vi "WF phase diversity_MATLAB_Correction_loop_AndorSDK_imq_NotOverwriteFolder.vi"() -> ()   [LabVIEW 2018]
uses:
  <userlib>/WaveKit.lib/Controls/Wavefront Corrector states - ONE.ctl
  <userlib>/WaveKit.lib/Classes/WavefrontCorrector/WavefrontCorrector.lvclass
  <userlib>/WaveKit.lib/Classes/WavefrontCorrectorSet/WavefrontCorrectorSet.lvclass
  <vilib>/Analysis/1siggen.llb/Ramp Pattern by Samples.vi
  <vilib>/Utility/file.llb/Read From Spreadsheet File (DBL).vi
  <vilib>/Analysis/1siggen.llb/Ramp Pattern by Delta.vi
  <vilib>/Analysis/NI_AALBase.lvlib
panel:
  in  "Tab Control":T1(tab)
  in  "Offset command file":path=path "D:/SystemAlignment/system_aberration_20200627.dat"
  in  "Initial haso file":path=path "D:/SystemAlignment/system_aberration_residual_20200627.has"
  out "# of Phase":i32
  in  "DM configuration file":path=path "C:/Program Files (x86)/Imagine Optic/Configuration Files/WaveFrontCorrector_mirao52-e_0326.dat"
  out "DM Initial State":T2[](array[typedef])
  out "DM ActuatorsNumber":i32
  out "Error out":errorcluster
  in  "Error in":errorcluster
  in  "EMCCD trigger port":tag="Dev1/port0/line0"
  in  "Cooler set to Temperature":i32=-60
  in  "Trigger":u32(ring)=1 items=["Internal", "External"]
  out "Return from CheckTimings":u32
  out "Calculated Exposure Value":sgl format="%.2f"
  out "Return from SetTemperature":u32
  out "Cooling":i32
  out "Return from Initialize":u32
  out "Detector X Pixels":i32
  out "Detector Y Pixels":i32
  in  "Initialize EMCCD?":bool=TRUE
  in  "Turn off EMCCD when finished?":bool
  in  "Initial Zer coeff":dbl[](array[numeric])=[0.2, 0.2]
  in  "Initial Zer index":dbl[](array[numeric])=[4.0, 5.0]
  out "Initial Zer coeff\nRandomly generated":dbl[](array[numeric])
  out "Initial Zer index (starting from 4)\nrandomly generated":dbl[](array[numeric])
  in  "aberration tolerance":dbl=0.1 format="%#_13g"
  in  "aberration threshold":dbl=0.25 format="%#_13g"
  in  "?":enum16{"input manually ", "randomly generated"}(ring)
  in  "max random order":i64=9
  in  "NOT YET: Data Acquisition Iteration #":i32=1
  in  "Zern index in 2":i32[](array[numeric])=[3, 4, 5, 6, 7, 8]
  in  "Zern coef in 2":sgl[](array[numeric])=[0.2, 0.5, 0.0, 0.0, 0.0, 0.0]
  in  "Zern index in 3":i32[](array[numeric])=[3, 4, 5, 6, 7, 8]
  in  "Zern coef in 3":sgl[](array[numeric])=[0.2, 0.0, 0.0, 0.0, 0.0, 0.0]
  in  "Zern index in 4":i32[](array[numeric])=[3, 4, 5, 6, 7, 8]
  in  "Zern coef in 4":sgl[](array[numeric])=[0.2, 0.0, 0.0, 0.0, 0.0, 0.0]
  in  "Zern index in 5":i32[](array[numeric])=[3, 4, 5, 6, 7, 8]
  in  "Zern coef in 5":sgl[](array[numeric])=[0.0, 0.0, 0.0, 0.0, 0.0, -0.2]
  in  "Andor Picture/notes save to path":path=path "D:/YD/test/test1"
  in  "base name":string="beads_test"
  in  "Pics/phase":dbl=2.0
  in  "camera exposure time (s)":string="0.02"
  in  "# of Phase":i32=5
  in  "COMMAND matrix path":path=path "D:/SystemAlignment/CM_20200711_0p5x6.aomc"
  in  "488 shutter":refnum<k7>(container)
  in  "?":bool
  out "phase diversity file name":string
  out "Corrected Picture name":string
  in  "Use GPU":bool=TRUE
  in  "Show Recon":bool=TRUE
  in  "Show Input":bool
  in  "Background Value":u32=290
  in  "Crop Size of image":u32=512
  in  "Gamma Value":dbl=1e-06
  in  "Iteration Number":u32=10
  in  "Zernike Order":u32=15
  in  "Number for average":u32=2
  in  "Run MATLAB or correction?":bool=TRUE
  in  "Keep Reconstructed Defocus component?":bool
  in  "Metrics Type":T3(ring)=enum."norm DCT  - spectral domain 3: 0~r0"
  in  "number of phase div image":dbl(ring)=2.0 items=["adding by step of 1 image"=1.0, "jump to 3 images"=0.9, "jump to 4 images"=2.0, "jump to 5 images"=2.9]
  # "priority:\n1, flip, done by Min on 20200731? \n2, organize\n3, new matlab PD code\n4. isolate shutdown\n\n\n\n2 PhasDiv first\nif not, take 3 more or start over 5\n\n??: random iteration work??\n\nadd preview"
  # "Cooler is off for testing"
  # "If Pics/phase is 2:\npicture order:\n\noffset+aberr *2\nphase diversity *8\n\nground truth *1\noffset+aberr *1\ncorrected *2 but the last one cannot be seen in imagej"
  # "Randomly Generate Initial Zernike, enter here:"
  # "Manually input, enter here:"
  # "Andor Camera Settings"
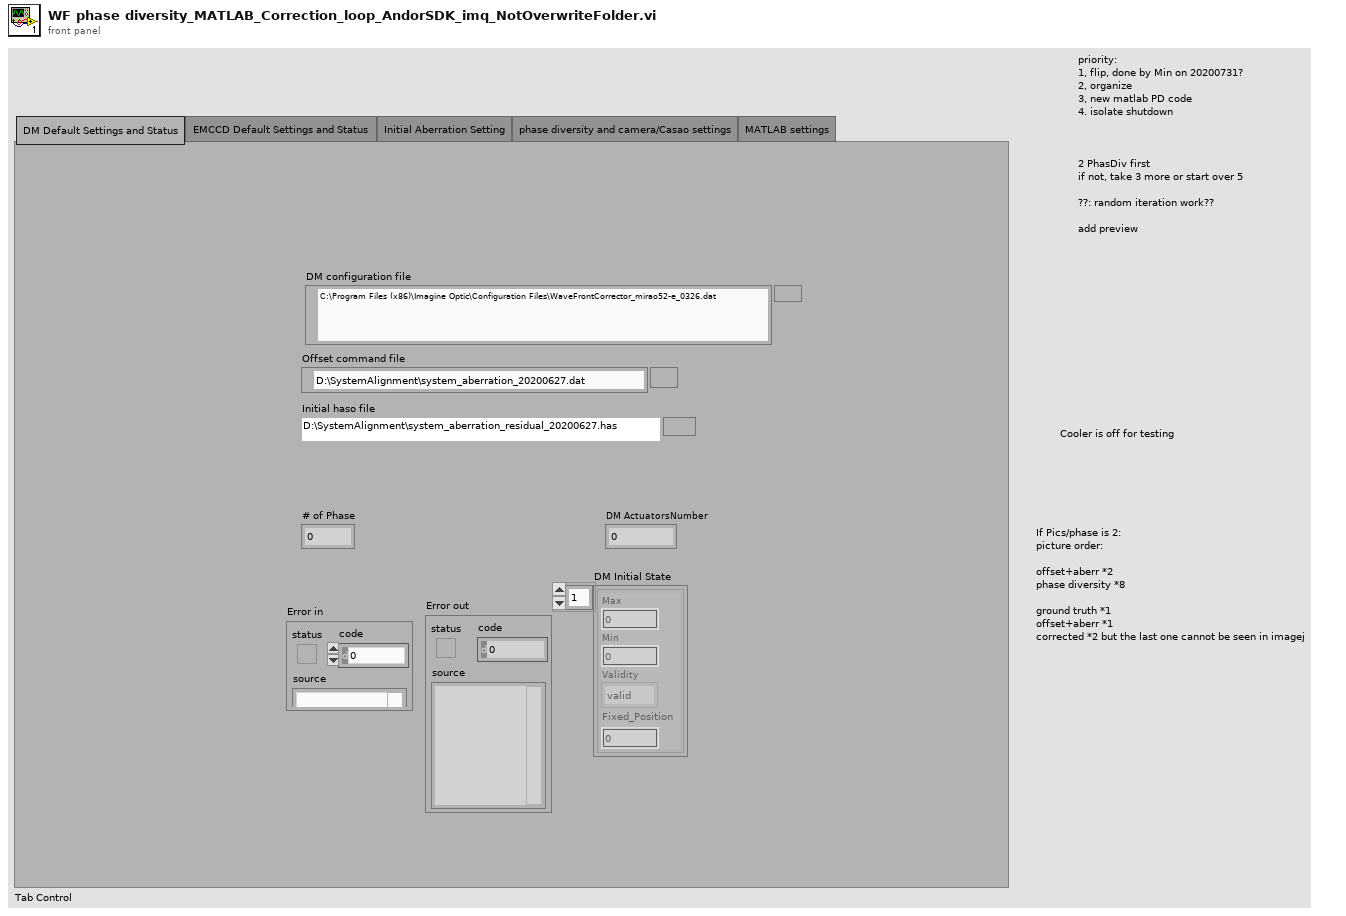
[diagram p1: front panel]
types:
  T1 = enum32{"DM Default Settings and Status", "EMCCD Default Settings and Status ", "Initial Aberration Setting", "phase diversity and camera/Casao settings", "MATLAB settings"}
  T2 = typedef "Wavefront Corrector states - ONE.ctl" = cluster{"Max":sgl, "Min":sgl, "Validity":enum16{"valid", "fixed", "invalid"}, "Fixed_Position":sgl}
  T3 = enum16{" ", "max intensity", "mean intensity", "RMS contrast", "sharpness - image domain", "sharpness - spectral domain 1: 0~r0", "sharpness - spectral domain 2: 0.1*r0~0.5*r0", "norm DCT  - spectral domain 3: 0~r0"}
  T4 = typedef "Error Code Enum typedef.ctl" = enum32{"N/A (0)", "DRV_ERROR_CODES", "DRV_SUCCESS", "DRV_VXDNOTINSTALLED", "DRV_ERROR_SCAN", "DRV_ERROR_CHECK_SUM", "DRV_ERROR_FILELOAD", "DRV_UNKNOWN_FUNC", "DRV_ERROR_VXD_INIT", "DRV_ERROR_ADDRESS", "DRV_ERROR_PAGELOCK", "DRV_ERROR_PAGEUNLOCK", "DRV_ERROR_BOARDTEST", "DRV_ERROR_ACK", "DRV_ERROR_UP_FIFO", "DRV_ERROR_PATTERN", "N/A (16)", "DRV_ACQUISITION_ERRORS", "DRV_ACQ_BUFFER", "DRV_ACQ_DOWNFIFO_FULL", "DRV_PROC_UNKONWN_INSTRUCTION", "DRV_ILLEGAL_OP_CODE", "DRV_KINETIC_TIME_NOT_MET", "DRV_ACCUM_TIME_NOT_MET", "DRV_NO_NEW_DATA", "N/A (25)", "DRV_SPOOLERROR", "N/A (27)", "N/A (28)", "N/A (29)", "N/A (30)", "N/A (31)", "N/A (32)", "DRV_TEMPERATURE_CODES", "DRV_TEMPERATURE_OFF", "DRV_TEMPERATURE_NOT_STABILIZED", "DRV_TEMPERATURE_STABILIZED", "DRV_TEMPERATURE_NOT_REACHED", "DRV_TEMPERATURE_OUT_RANGE", "DRV_TEMPERATURE_NOT_SUPPORTED", "DRV_TEMPERATURE_DRIFT", "N/A (41)", "N/A (42)", "N/A (43)", "N/A (44)", "N/A (45)", "N/A (46)", "N/A (47)", "N/A (48)", "DRV_GENERAL_ERRORS", "DRV_INVALID_AUX", "DRV_COF_NOTLOADED", "DRV_FPGAPROG", "DRV_FLEXERROR", "DRV_GPIBERROR", "N/A (55)", "N/A (56)", "N/A (57)", "N/A (58)", "N/A (59)", "N/A (60)", "N/A (61)", "N/A (62)", "N/A (63)", "DRV_DATATYPE", "DRV_DRIVER_ERRORS", "DRV_P1INVALID", "DRV_P2INVALID", "DRV_P3INVALID", "DRV_P4INVALID", "DRV_INIERROR", "DRV_COFERROR", "DRV_ACQUIRING", "DRV_IDLE", "DRV_TEMPCYCLE", "DRV_NOT_INITIALIZED", "DRV_P5INVALID", "DRV_P6INVALID", "DRV_INVALID_MODE", "DRV_INVALID_FILTER", "DRV_I2CERRORS", "DRV_I2CDEVNOTFOUND", "DRV_I2CTIMEOUT", "DRV_P7INVALID", "N/A (84)", "N/A (85)", "N/A (86)", "N/A (87)", "N/A (88)", "N/A (89)", "DRV_IOCERROR", "DRV_VRMVERSIONERROR"}
  T5 = typedef "NI_Matrix.lvlib/RealMatrix.ctl" = dbl[][]
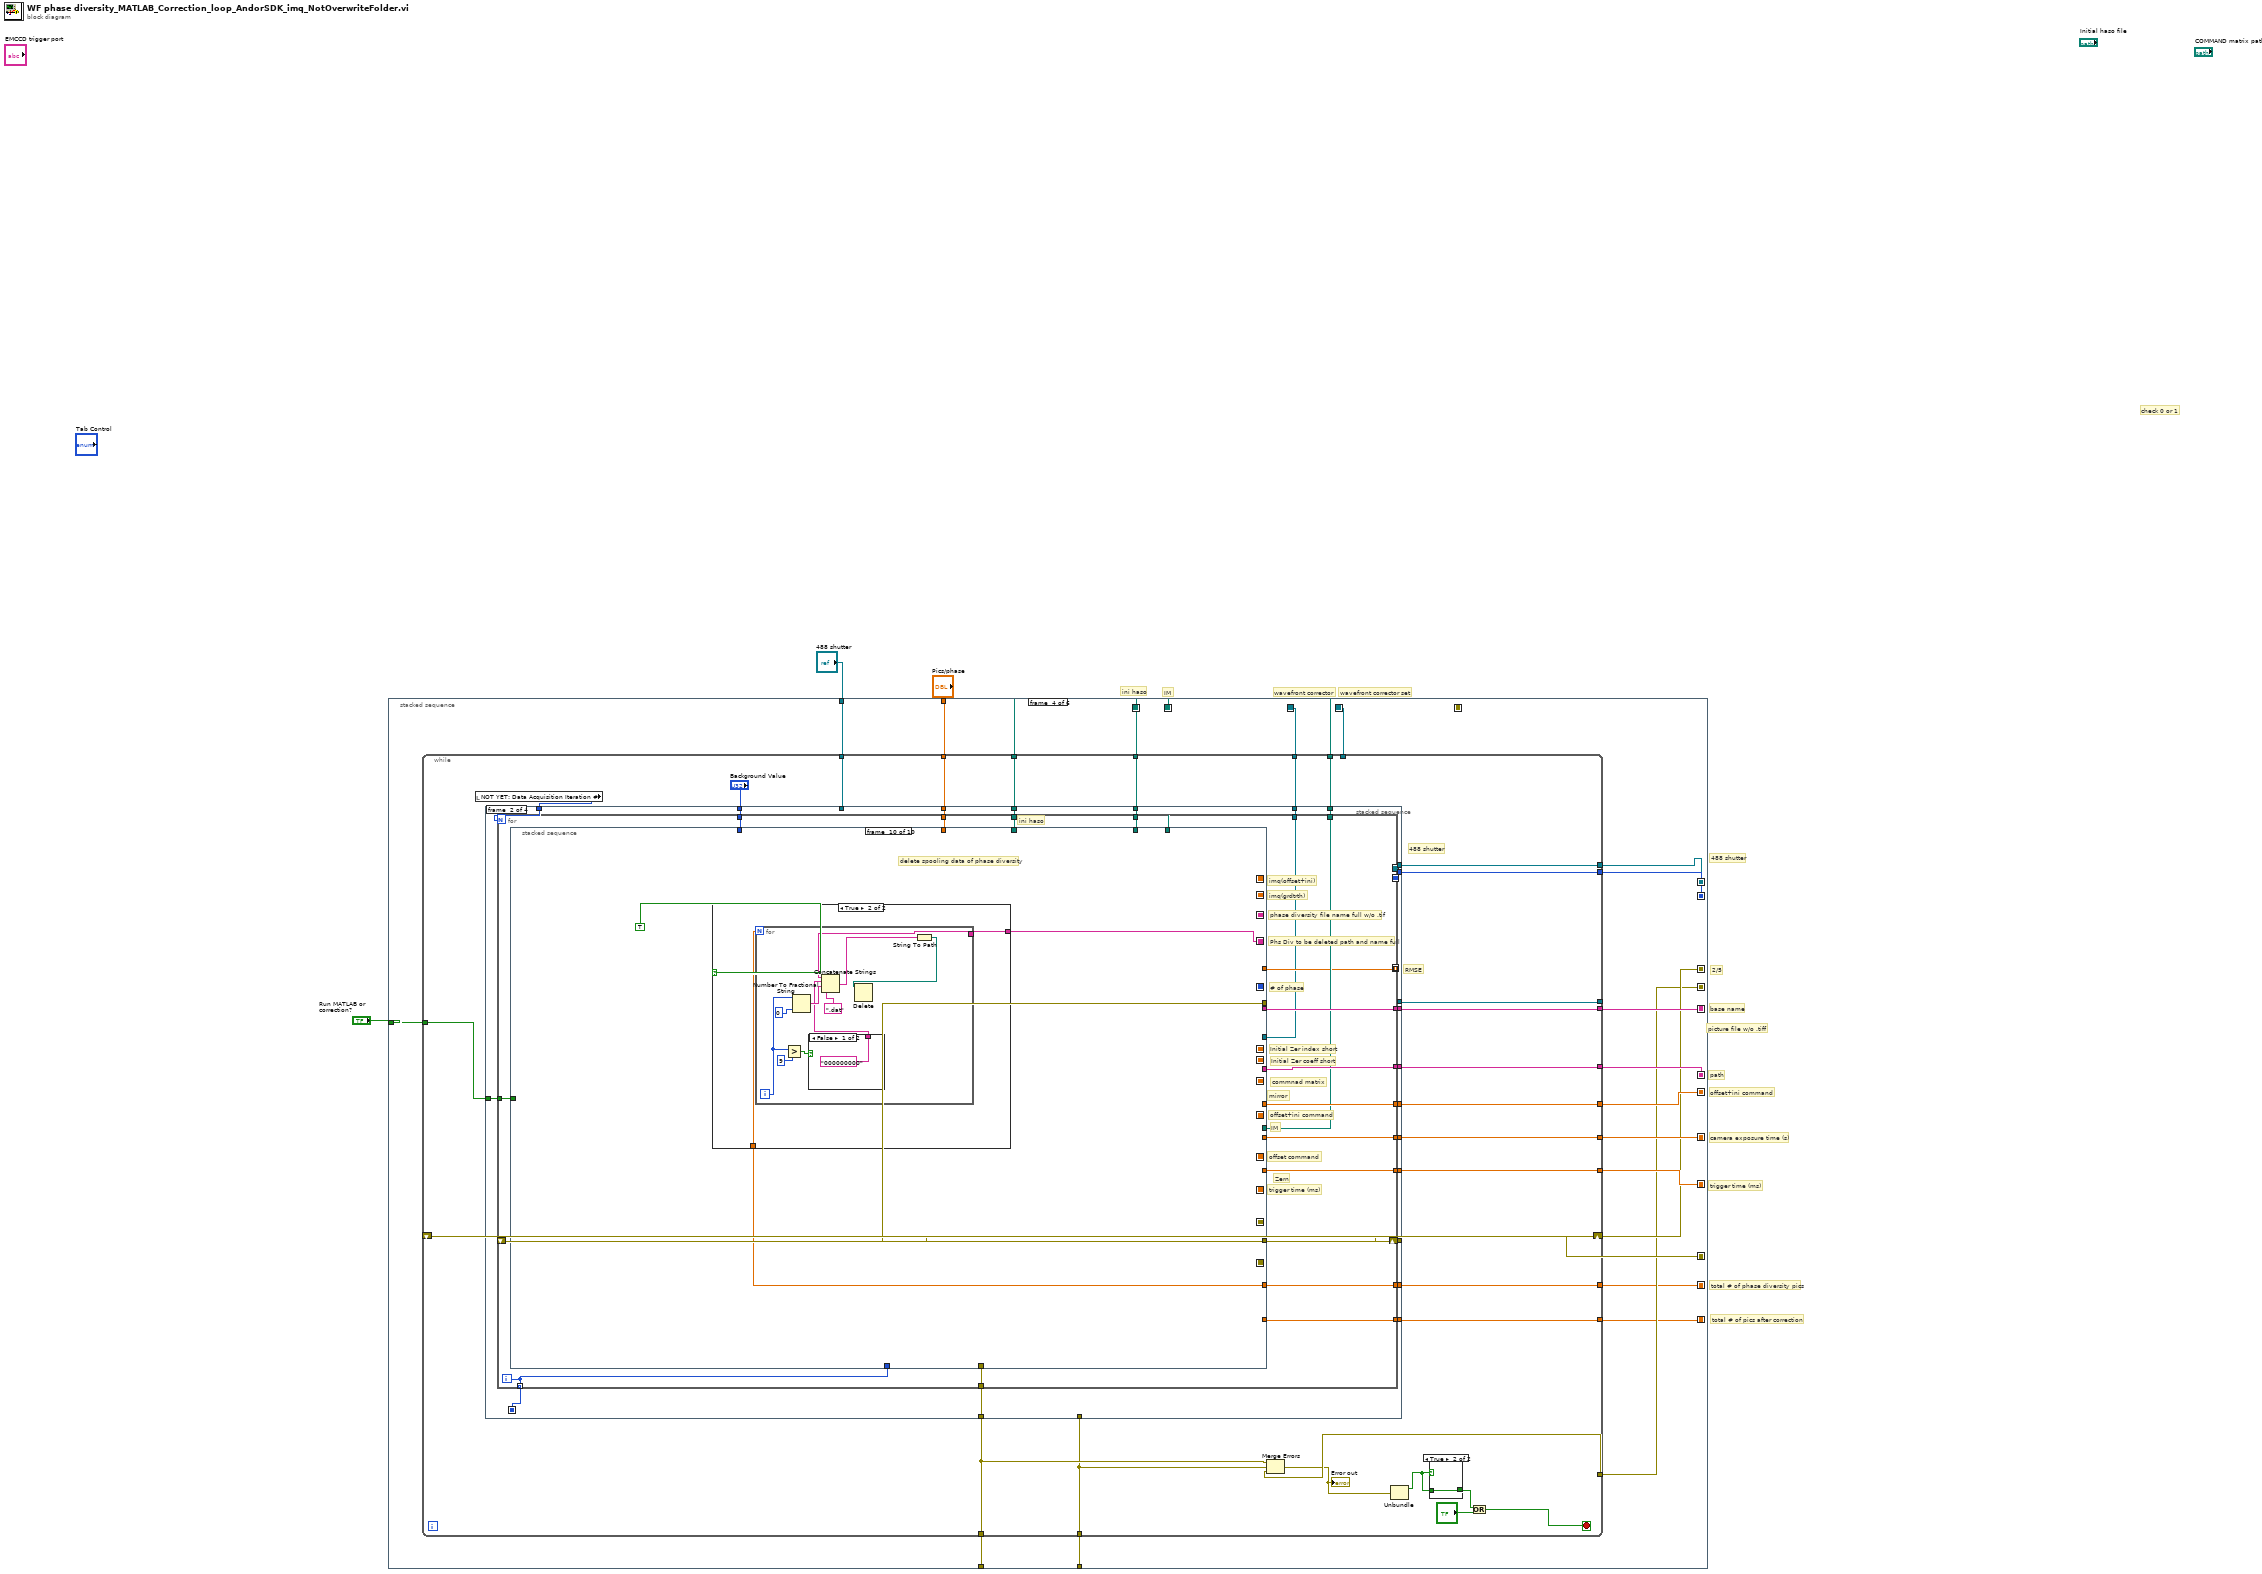
[diagram p0: block diagram]
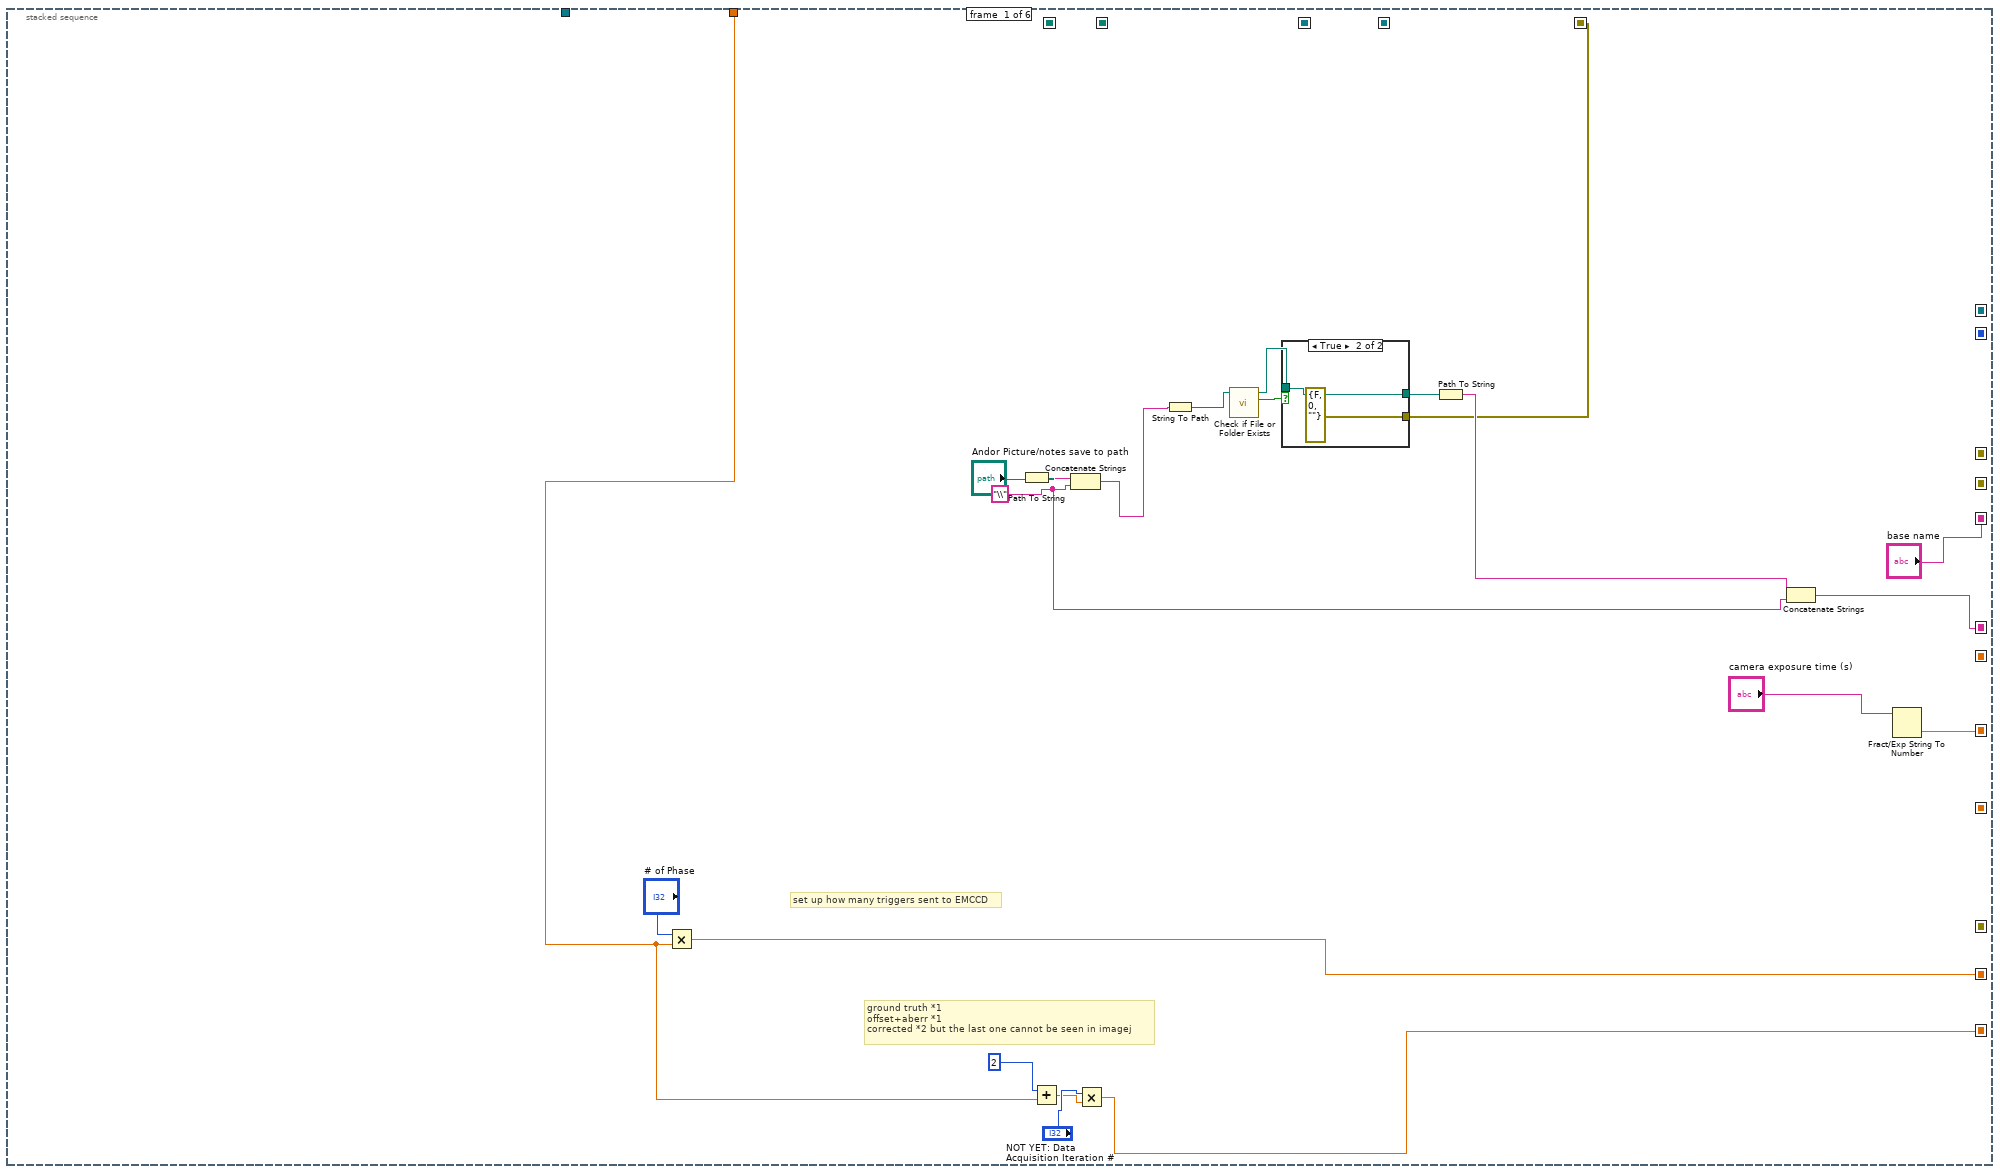
[diagram p2: hidden frame]
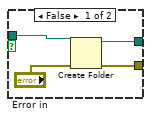
[diagram p3: hidden frame]
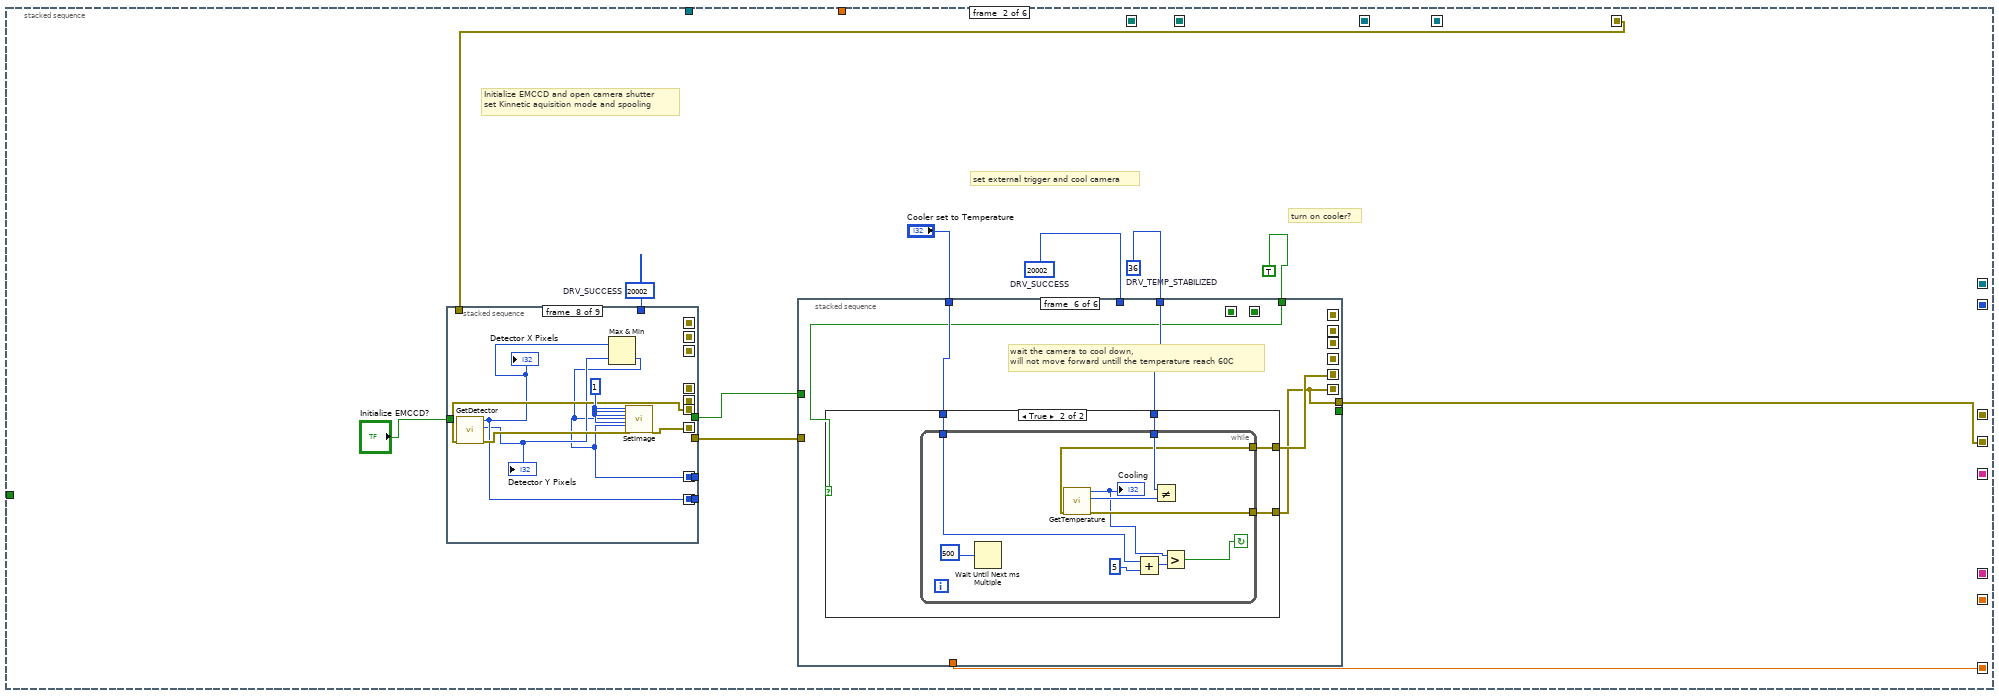
[diagram p4: hidden frame]
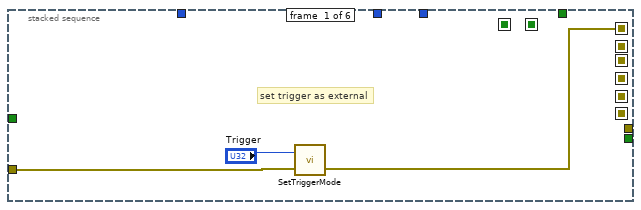
[diagram p5: hidden frame]
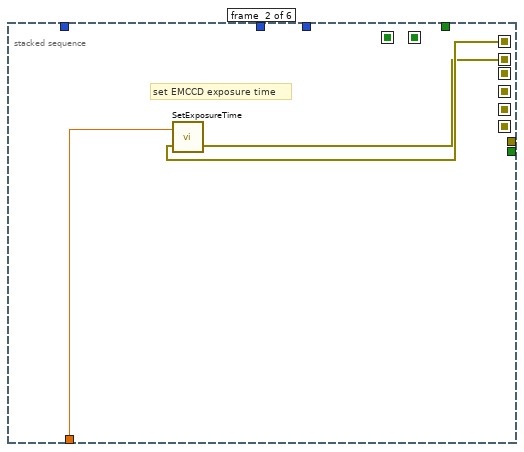
[diagram p6: hidden frame]
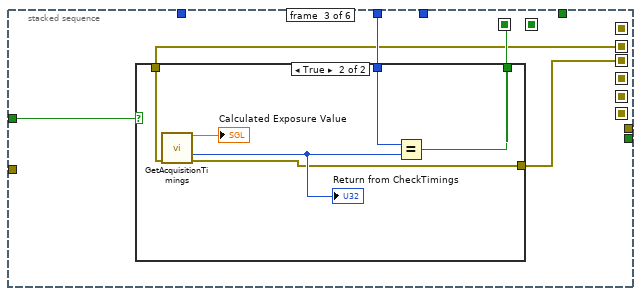
[diagram p7: hidden frame]
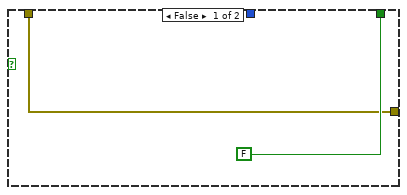
[diagram p8: hidden frame]
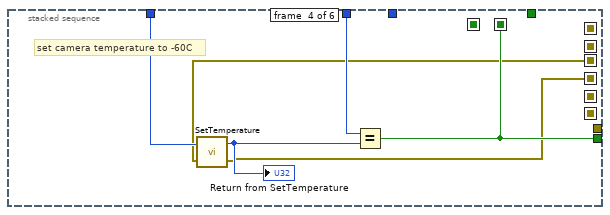
[diagram p9: hidden frame]
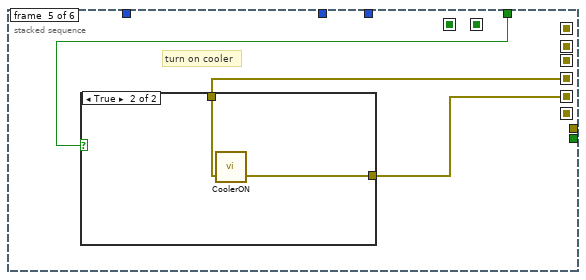
[diagram p10: hidden frame]
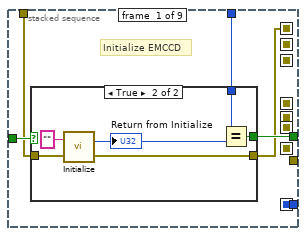
[diagram p13: hidden frame]
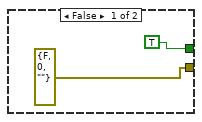
[diagram p14: hidden frame]
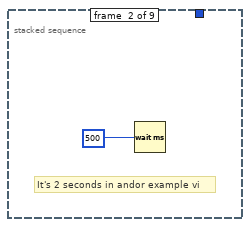
[diagram p15: hidden frame]
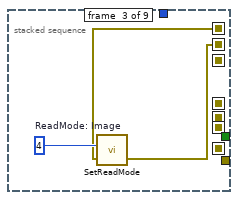
[diagram p16: hidden frame]
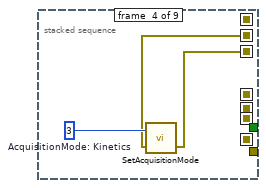
[diagram p17: hidden frame]
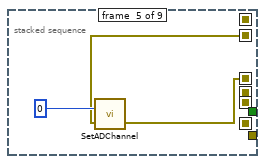
[diagram p18: hidden frame]
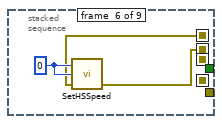
[diagram p19: hidden frame]
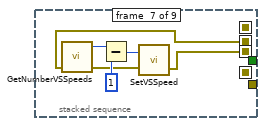
[diagram p20: hidden frame]
diagram:
  # "2/5"
  # "total # of phase diversity pics"
  # "picture file w/o .tiff"
  # "total # of pics after correction"
  # "wavefront corrector set"
  # "wavefront corrector"
  # "488 shutter"
  # "trigger time (ms)"
  # "offset+ini command"
  # "camera exposure time (s)"
  # "IM"
  # "ini haso"
  # "path"
  # "base name"
  # "check 0 or 1"
  n1 = stacked-sequence {
    seq-local: [w5 _ _ _ _ _] -> [_ _ _ w174 _ _]
    seq-local: ["base name" _ _ _ _ _] -> [_ _ _ w173 _ _]
    seq-local: [_ _ w154 _ _ _] -> [_ _ _ w155 _ _]
    seq-local: [_ _ w153 _ _ _] -> [_ _ _ w168 _ _]
    seq-local: [w19 _ _ _ _ _] -> [_ w34 _ w172 _ _]
    seq-local: [_ _ w139 _ _ _] -> [_ _ _ w160 _ _]
    seq-local: [_ _ _ w171 _ _] -> [_ _ _ _ _ _]
    seq-local: [_ _ _ w170 _ _] -> [_ _ _ _ _ _]
    seq-local: [_ _ _ w169 _ _] -> [_ _ _ _ _ w788]
    seq-local: [_ _ _ w163 _ _] -> [_ _ _ _ _ _]
    seq-local: [_ _ _ w166 _ _] -> [_ _ _ _ _ _]
    seq-local: [_ _ w138 _ _ _] -> [_ _ _ w161 _ w790]
    seq-local: [_ _ w137 _ _ _] -> [_ _ _ w159 _ w789]
    seq-local: [w16 _ _ _ _ _] -> [_ _ _ w156 _ _]
    seq-local: [_ w35 _ _ _ _] -> [_ _ w136 w158 _ _]
    seq-local: [w15 _ _ _ _ _] -> [_ _ _ w157 _ _]
    seq-local: [w4 _ _ _ _ _] -> [_ w31 _ _ _ _]
    tunnel: "Pics/phase" -> [w13 _ _ w175 _ _]
    tunnel: "Run MATLAB or correction?" -> [_ _ _ w167 _ _]
    tunnel: [_ _ _ w165 _ _] -> _
    tunnel: [_ _ _ w164 _ _] -> _
    tunnel: "488 shutter" -> [_ _ _ w162 _ w791]
    frame #0 {
      w6 = "\\"
      # "set up how many triggers sent to EMCCD"
      # "ground truth *1\noffset+aberr *1\ncorrected *2 but the last one cannot be seen in imagej"
      n2 = Multiply(x="# of Phase", y=w13) -> (x*y=w15:dbl)
      n3 = Path To String(path="Andor Picture/notes save to path") -> (string=w21:string)
      n4 = Add(x=2, y=w13) -> (x+y=w17:dbl)
      n5 = Concatenate Strings(w21, w6) -> (w8:string)
      n6 = Multiply(x="NOT YET: Data Acquisition Iteration #", y=w17) -> (x*y=w16:dbl)
      n7 = String To Path(string=w8) -> (path=w12:path)
      n8 = call <vilib>:"Check if File or Folder Exists.vi"("path"=w12) -> ("file or folder exists?"=w10:bool, "dup path"=w11:path)  [unwired: 8 in, 1 out]
      n9 = case shown="True" w10 {
        tunnel: w11 -> [w28 w30]
        tunnel: [w27 w30] -> w9
        tunnel: [w25 errorcluster {"status"=FALSE, "code"=0, "source"=""} ("Error in 3")] -> w4
        frame False {
          n10 = Create Folder(path (use dialog)=w28, error in="Error in") -> (created path=w27:path, error out=w25:errorcluster)  [unwired: 1 in, 1 out]
        }
        frame True {
        }
      }
      n11 = Path To String(path=w9) -> (string=w7:string)
      n12 = Concatenate Strings(w7, w6) -> (w5:string)
      n13 = Fract/Exp String To Number(string="camera exposure time (s)") -> (number=w19:dbl)  [unwired: 3 in, 1 out]
    }
    frame #1 {
      w37 = 36  # DRV_TEMP_STABILIZED
      w39 = 20002  # DRV_SUCCESS
      w41 = 20002  # DRV_SUCCESS
      # "turn on cooler?"
      # "set external trigger and cool camera"
      # "Initialize EMCCD and open camera shutter\nset Kinnetic aquisition mode and spooling"
      n14 = stacked-sequence {
        seq-local: [_ _ _ _ _ _ _ w125 _] -> [_ _ _ _ _ _ _ _ _]
        seq-local: [_ _ _ _ _ _ _ w127 _] -> [_ _ _ _ _ _ _ _ _]
        seq-local: [w95 _ _ _ _ _ _ _ _] -> [_ _ w108 _ _ _ _ _ _]
        seq-local: [_ _ w107 _ _ _ _ _ _] -> [_ _ _ w111 _ _ _ _ _]
        seq-local: [_ _ _ w110 _ _ _ _ _] -> [_ _ _ _ w113 _ _ _ _]
        seq-local: [_ _ _ _ w114 _ _ _ _] -> [_ _ _ _ _ w117 _ _ _]
        seq-local: [_ _ _ _ _ w116 _ _ _] -> [_ _ _ _ _ _ w121 _ _]
        seq-local: [_ _ _ _ _ _ w119 _ _] -> [_ _ _ _ _ _ _ w130 _]
        seq-local: [_ _ _ _ _ _ _ w128 _] -> [_ _ _ _ _ _ _ _ w133]
        tunnel: w41 -> [w97 _ _ _ _ _ _ _ _]
        tunnel: [w96 _ _ _ _ _ _ _ _] -> w40
        tunnel: [_ _ _ _ _ _ _ w125 _] -> _
        tunnel: [_ _ _ _ _ _ _ w127 _] -> _
        tunnel: [_ _ _ _ _ _ _ _ w132] -> w36
        tunnel: "Initialize EMCCD?" -> [w94 _ _ _ _ _ _ _ _]
        tunnel: w31 -> [w93 _ _ _ _ _ _ _ _]
        frame #0 {
          # "Initialize EMCCD"
          n15 = case shown="True" w94 {
            tunnel: w97 -> [_ w103]
            tunnel: [TRUE w102] -> w96
            tunnel: [errorcluster {"status"=FALSE, "code"=0, "source"=""} ("Error in 2") w101] -> w95
            tunnel: w93 -> [_ w100]
            frame False {
            }
            frame True {
              n16 = call <userlib>:"Initialize.vi"("error in (no error)"=w100, "directory (\"\")"="" ("directory (\"\")")) -> ("error out"=w101:errorcluster, "DLL error code"=w105:u32)
              "Return from Initialize" <- w105
              n17 = Equal?(x=w103, y=w105) -> (x = y?=w102:bool)
            }
          }
        }
        frame #1 {
          # "It's 2 seconds in andor example vi"
          n18 = Wait (ms)(milliseconds to wait=u32 500) -> ()  [unwired: 1 out]
        }
        frame #2 {
          w109 = u16 4  # ReadMode: Image
          n19 = call <userlib>:"SetReadMode.vi"("error in (no error)"=w108, "mode"=w109) -> ("error out"=w107:errorcluster)  [unwired: 1 out]
        }
        frame #3 {
          w112 = u16 3  # AcquisitionMode: Kinetics
          n20 = call <userlib>:"SetAcquisitionMode.vi"("error in (no error)"=w111, "mode"=w112) -> ("error out"=w110:errorcluster)  [unwired: 1 out]
        }
        frame #4 {
          n21 = call <userlib>:"SetADChannel.vi"("error in (no error)"=w113, "channel"=0) -> ("error out"=w114:errorcluster)  [unwired: 1 out]
        }
        frame #5 {
          w118 = 0
          n22 = call <userlib>:"SetHSSpeed.vi"("error in (no error)"=w117, "index"=w118, "type"=w118) -> ("error out"=w116:errorcluster)  [unwired: 1 in, 1 out]
        }
        frame #6 {
          n23 = call <userlib>:"GetNumberVSSpeeds.vi"("error in (no error)"=w121) -> ("error out"=w120:errorcluster, "number"=w124:i32)  [unwired: 2 in, 1 out]
          n24 = Subtract(x=w124, y=1) -> (x-y=w122:i32)
          n25 = call <userlib>:"SetVSSpeed.vi"("error in (no error)"=w120, "index"=w122) -> ("error out"=w119:errorcluster)  [unwired: 1 out]
        }
        frame #7 {
          w131 = 1
          n26 = call <userlib>:"GetDetector.vi"("error in (no error)"=w130) -> ("error out"=w129:errorcluster, "ypixels"=w126:i32, "xpixels"=w127:i32)  [unwired: 3 in, 1 out]
          "Detector Y Pixels" <- w126
          "Detector X Pixels" <- w127
          n27 = Max & Min(x=w127, y=w126) -> (min(x,y)=w125:i32)  [unwired: 1 out]
          n28 = call <userlib>:"SetImage.vi"("hbin"=w131, "vbin"=w131, "hstart"=w131, "hend"=w125, "vstart"=w131, "vend"=w125, "error in (no error)"=w129) -> ("error out"=w128:errorcluster)  [unwired: 19 in, 1 out]
        }
        frame #8 {
          w134 = 0
          w135 = 1
          n29 = call <userlib>:"SetShutter.vi"("type"=w135, "mode"=w135, "closingtime"=w134, "openingtime"=w134, "error in (no error)"=w133) -> ("error out"=w132:errorcluster)  [unwired: 9 in, 1 out]
        }
      }
      n30 = stacked-sequence {
        seq-local: [_ _ w50 _ _ _] -> [_ _ _ _ _ _]
        seq-local: [_ _ _ w63 _ _] -> [_ _ _ _ _ _]
        seq-local: [w42 _ _ _ _ _] -> [_ w47 _ _ _ _]
        seq-local: [_ w46 _ _ _ _] -> [_ _ w49 _ _ _]
        seq-local: [_ _ w48 _ _ _] -> [_ _ _ w62 _ _]
        seq-local: [_ _ _ w61 _ _] -> [_ _ _ _ w69 _]
        seq-local: [_ _ _ _ w68 _] -> [_ _ _ _ _ w75]
        seq-local: [_ _ _ _ _ w73] -> [_ _ _ _ _ _]
        tunnel: w39 -> [_ _ w52 w66 _ _]
        tunnel: "Cooler set to Temperature" -> [_ _ _ w64 _ w76]
        tunnel: w37 -> [_ _ _ _ _ w77]
        tunnel: [_ _ _ w63 _ _] -> _
        tunnel: w40 -> [_ _ w51 _ _ _]
        tunnel: w36 -> [w43 _ _ _ _ _]
        tunnel: [_ _ _ _ _ w73] -> w35
        tunnel: w34 -> [_ w45 _ _ _ _]
        tunnel: TRUE -> [_ _ _ _ w67 w74]
        frame #0 {
          # "set trigger as external"
          n31 = call <userlib>:"SetTriggerMode.vi"("error in (no error)"=w43, "mode"="Trigger") -> ("error out"=w42:errorcluster)  [unwired: 1 out]
        }
        frame #1 {
          # "set EMCCD exposure time"
          n32 = call <userlib>:"SetExposureTime.vi"("error in (no error)"=w47, "time"=w45) -> ("error out"=w46:errorcluster)  [unwired: 1 out]
        }
        frame #2 {
          n33 = case shown="True" w51 {
            tunnel: w52 -> [_ w58]
            tunnel: [FALSE w60] -> w50
            tunnel: w49 -> [w53 w56]
            tunnel: [w53 w55] -> w48
            frame False {
            }
            frame True {
              n34 = call <userlib>:"GetAcquisitionTimings.vi"("error in (no error)"=w56) -> ("exposure"=→"Calculated Exposure Value":sgl, "DLL error code"=w57:u32, "error out"=w55:errorcluster)  [unwired: 10 in, 2 out]
              "Return from CheckTimings" <- w57
              n35 = Equal?(x=w58, y=w57) -> (x = y?=w60:bool)
            }
          }
        }
        frame #3 {
          # "set camera temperature to -60C"
          n36 = call <userlib>:"SetTemperature.vi"("error in (no error)"=w62, "temperature"=w64) -> ("error out"=w61:errorcluster, "DLL error code"=w65:u32)
          "Return from SetTemperature" <- w65
          n37 = Equal?(x=w66, y=w65) -> (x = y?=w63:bool)
        }
        frame #4 {
          # "turn on cooler"
          n38 = case shown="True" w67 {
            tunnel: w69 -> [w70 w72]
            tunnel: [w70 w71] -> w68
            frame False {
            }
            frame True {
              n39 = call <userlib>:"CoolerON.vi"("error in (no error)"=w72) -> ("error out"=w71:errorcluster)  [unwired: 1 in, 1 out]
            }
          }
        }
        frame #5 {
          # "wait the camera to cool down,\nwill not move forward untill the temperature reach 60C"
          n40 = case shown="True" w74 {
            tunnel: w77 -> [_ w82]
            tunnel: w76 -> [_ w81]
            tunnel: w75 -> [w78 w80]
            tunnel: [w78 w79] -> w73
            frame False {
            }
            frame True {
              n41 = while {
                tunnel: w82 -> [w91]
                tunnel: w81 -> [w86]
                tunnel: w80 -> [w89]
                tunnel: [w88] -> w79
                stop <- w83 continue-if-true
                n42 = Wait Until Next ms Multiple(millisecond multiple=u32 500) -> ()  [unwired: 1 out]
                n43 = call <userlib>:"GetTemperature.vi"("error in (no error)"=w89) -> ("error out"=w88:errorcluster, "status"=w90:T4, "temperature"=w84:i32)  [unwired: 3 in, 1 out]
                "Cooling" <- w84
                n44 = Add(x=w86, y=5) -> (x+y=w85:i32)
                n45 = Not Equal?(x=w91, y=w90) -> ()  [unwired: 1 out]
                n46 = Greater?(x=w84, y=w85) -> (0:w83:bool)
              }
            }
          }
        }
      }
    }
    frame #2 {
      # "Initialize CASAO"
      n47 = call <userlib>:"LVClass_WavefrontCorrectorSet ctor.vi"("WavefrontCorrectorSet in"=refnum<class "WavefrontCorrectorSet.lvclass"> refnum, "PathToWavefrontCorrectorSetupFile"="DM configuration file", "error in (no error)"=w136) -> ("WavefrontCorrectorSet out"=w143:refnum<class "WavefrontCorrectorSet.lvclass">, "error out"=w152:errorcluster)  [unwired: 11 in]
      n48 = call <userlib>:"LVClass_WavefrontCorrector ctor.vi"("WavefrontCorrector in"=refnum<class "WavefrontCorrector.lvclass"> refnum, "PathToWavefrontCorrectorSetupFile"="DM configuration file", "error in (no error)"=w152) -> ("WavefrontCorrector out"=w147:refnum<class "WavefrontCorrector.lvclass">, "error out"=w146:errorcluster)  [unwired: 11 in]
      n49 = call <userlib>:"LVClass_WavefrontCorrector Init.vi"("WavefrontCorrector in"=w147, "set_init_state_from_config_file"=TRUE, "error in (no error)"=w146) -> ("WavefrontCorrector out"=w141:refnum<class "WavefrontCorrector.lvclass">, "error out"=w145:errorcluster)  [unwired: 11 in]
      n50 = call <userlib>:"LVClass_WavefrontCorrectorSet get nb of actuators.vi"("WavefrontCorrectorSet in"=w143, "error in (no error)"=w145) -> ("WavefrontCorrectorSet out"=w137:refnum<class "WavefrontCorrectorSet.lvclass">, "ActuatorsNumber"=→"DM ActuatorsNumber":i32, "error out"=w142:errorcluster)  [unwired: 11 in]
      n51 = call <userlib>:"LVClass_WavefrontCorrector Get Current Preferences.vi"("WavefrontCorrector in"=w141, "error in (no error)"=w142) -> ("WavefrontCorrector out"=w138:refnum<class "WavefrontCorrector.lvclass">, "Mirror preferences.Wavefront Corrector State"=→"DM Initial State":T2[], "error out"=w139:errorcluster)  [unwired: 10 in, 1 out]
      n52 = local read "COMMAND matrix path"() -> (w153:path)
      n53 = local read "Initial haso file"() -> (w154:path)
    }
    frame #3 {
      n54 = while {
        tunnel: w175 -> [w204]
        tunnel: w174 -> [w203]
        tunnel: w173 -> [w202]
        tunnel: w155 -> [w201]
        tunnel: w172 -> [w200]
        tunnel: [w198] -> w171
        tunnel: [w197] -> w170
        tunnel: w168 -> [w195]
        tunnel: w167 -> [w194]
        tunnel: [w193] -> w166
        tunnel: [w192] -> _
        tunnel: [w190] -> w165
        tunnel: [w191] -> w164
        shift-right: [w196] -> w169
        shift-left: w160 -> [w199]
        tunnel: [w189] -> w163
        tunnel: w162 -> [w188]
        tunnel: w161 -> [w187]
        tunnel: w159 -> [_]
        tunnel: w158 -> [w185]
        tunnel: w157 -> [w179]
        tunnel: w156 -> [w178]
        tunnel: w155 -> [w176]
        stop <- w181 stop-if-true
        # "488 shutter"
        # "RMSE"
        n55 = local read "NOT YET: Data Acquisition Iteration #"() -> (w186:i32)
        n56 = stacked-sequence {
          seq-local: [_ w222 _ _] -> [_ _ _ w780]
          seq-local: [_ w221 _ _] -> [_ _ _ _]
          seq-local: [w209 _ _ _] -> [_ _ w776 _]
          seq-local: [w210 _ _ _] -> [_ _ w775 _]
          tunnel: w204 -> [_ w234 _ _]
          tunnel: w203 -> [_ w233 _ w779]
          tunnel: w202 -> [_ w232 _ w778]
          tunnel: w201 -> [_ w231 _ _]
          tunnel: w200 -> [_ w230 _ _]
          tunnel: w199 -> [_ w229 _ _]
          tunnel: [_ w228 _ _] -> w198
          tunnel: [_ w227 _ _] -> w197
          tunnel: [_ w226 _ _] -> w196
          tunnel: w195 -> [_ w225 _ _]
          tunnel: w194 -> [_ w224 _ _]
          tunnel: w186 -> [_ w223 _ _]
          tunnel: [_ _ w774 _] -> w192
          tunnel: [_ _ w773 _] -> w193
          tunnel: [_ _ _ w777] -> w190
          tunnel: [_ w220 _ _] -> w191
          tunnel: [w209 _ _ _] -> w189
          tunnel: w188 -> [w208 _ _ _]
          tunnel: w187 -> [_ w219 _ _]
          tunnel: w179 -> [_ w218 _ _]
          tunnel: w178 -> [_ w217 _ _]
          tunnel: "Background Value" -> [_ w216 _ _]
          tunnel: w176 -> [_ w215 _ _]
          frame #0 {
            # "open the shutter of 488nm laser"
            n57 = property class="MG17Motor"(reference=w208, "HWSerialNum"=85819115.0) -> (reference out=w214:refnum<k7>)  [unwired: 1 in, 1 out]
            n58 = invoke class="MG17Motor" method="StartCtrl"(reference=w214) -> (reference out=w212:refnum<k7>)  [unwired: 2 in, 2 out]
            n59 = invoke class="MG17Motor" method="SC_Enable"(reference=w212, "lChanID"=0) -> (reference out=w209:refnum<k7>, "lChanID"=w210:i32)  [unwired: 2 in, 2 out]
          }
          frame #1 {
            n60 = for {
              N: w223 -> [_]
              tunnel: w234 -> [w253]
              tunnel: w233 -> [w252]
              tunnel: w232 -> [w251]
              tunnel: w231 -> [w250]
              tunnel: w230 -> [w249]
              tunnel: [w247] -> w228
              tunnel: [w246] -> w227
              tunnel: w225 -> [w244]
              tunnel: w224 -> [w243]
              shift-right: [w245] -> w226
              shift-left: w229 -> [w248]
              tunnel: [w242] -> w222 mode=indexing
              tunnel: [w241] -> w221 mode=indexing
              tunnel: [w240] -> w220
              tunnel: w219 -> [w239]
              tunnel: w218 -> [w238]
              tunnel: w217 -> [w237]
              tunnel: w216 -> [w236]
              tunnel: w215 -> [w235]
              i -> [w241]
              # "imq(grdtrth)"
              # "imq(offset+ini)"
              # "Phs Div to be deleted path and name full"
              # "phase diversity file name full w/o .tif"
              # "# of phase"
              # "trigger time (ms)"
              # "offset+ini command"
              # "Initial Zer coeff short"
              # "Initial Zer index short"
              # "mirror"
              # "Zern"
              # "commnad matrix"
              # "ini haso"
              # "IM"
              # "offset command"
              n61 = stacked-sequence {
                seq-local: [_ w265 _ _ _ _ _ _ _ _] -> [_ _ w285 _ w413 _ _ w472 w525 _]
                seq-local: [_ _ w283 _ _ _ _ _ _ _] -> [_ _ _ _ w412 _ _ _ w527 _]
                seq-local: [_ _ w281 _ _ _ _ _ _ _] -> [_ _ _ _ w411 _ _ _ _ _]
                seq-local: [_ _ w274 _ _ _ _ _ _ _] -> [_ _ _ _ w408 _ _ _ _ _]
                seq-local: [w256 _ _ _ _ _ _ _ _ _] -> [_ _ w271 _ _ _ _ _ _ _]
                seq-local: [w255 _ _ _ _ _ _ _ _ _] -> [_ _ w270 _ _ _ _ _ _ _]
                seq-local: [_ _ w269 _ _ _ _ _ _ _] -> [_ _ _ _ _ _ _ w474 w531 _]
                seq-local: [_ _ _ _ w407 _ _ _ _ _] -> [_ _ _ _ _ w457 _ w477 w518 _]
                seq-local: [_ _ _ _ w406 _ _ _ _ _] -> [_ _ _ _ _ _ _ _ w529 _]
                seq-local: [_ _ _ _ _ _ w460 _ _ _] -> [_ _ _ _ _ _ _ _ w521 _]
                seq-local: [_ _ _ w400 _ _ _ _ _ _] -> [_ _ _ _ _ _ _ _ _ w758]
                seq-local: [_ _ _ _ _ _ _ w473 _ _] -> [_ _ _ _ _ _ _ _ _ _]
                seq-local: [_ _ _ _ _ _ _ w471 _ _] -> [_ _ _ _ _ _ _ _ w519 _]
                tunnel: w253 -> [_ _ w278 _ w416 _ _ _ w530 _]
                tunnel: w252 -> [_ _ w279 w403 w415 _ w468 w480 w533 _]
                tunnel: w251 -> [_ _ w280 w402 w414 _ w470 w479 w534 _]
                tunnel: w250 -> [_ _ w277 _ _ _ _ _ w516 _]
                tunnel: w244 -> [_ _ w276 _ w410 _ _ _ _ _]
                tunnel: w249 -> [_ _ _ _ w409 _ _ _ _ _]
                tunnel: w248 -> [_ _ w275 _ _ _ _ _ _ _]
                tunnel: [_ _ _ _ w406 _ _ _ _ _] -> w245
                tunnel: [_ _ w269 _ _ _ _ _ _ _] -> w247
                tunnel: [_ _ _ _ w407 _ _ _ _ _] -> w246
                tunnel: w244 -> [_ _ _ _ _ _ _ _ w532 _]
                tunnel: w243 -> [_ _ _ _ _ _ _ _ w528 _]
                tunnel: w241 -> [_ _ w268 w399 _ _ w469 w478 w517 _]
                tunnel: [_ _ _ _ _ _ _ _ w526 _] -> w242
                tunnel: [_ _ _ _ _ _ _ _ w524 _] -> w240
                tunnel: w239 -> [_ _ _ _ w405 _ _ w476 w523 _]
                tunnel: w238 -> [_ _ _ w404 _ _ _ _ _ w756]
                tunnel: w237 -> [_ _ _ _ _ _ _ _ w522 _]
                tunnel: w236 -> [_ _ _ _ _ _ _ w475 w520 _]
                tunnel: w235 -> [_ _ _ _ _ _ _ _ w515 _]
                frame #0 {
                  # "generate initial aberration (aberr to correct)"
                  n62 = case shown="\"randomly generated\"" "?" {
                    tunnel: ["Initial Zer index" w262] -> w256
                    tunnel: ["Initial Zer coeff" w261] -> w255
                    tunnel: "max random order" -> [_ w260]
                    frame "input manually " {
                    }
                    frame "randomly generated" {
                      # "generate random zernike index and coefficient arrays"
                      n63 = call "Random Aberration Array Generator.vi"("max random order"=w260, "aberration tolerance"="aberration tolerance", "aberration threshold"="aberration threshold") -> ("Zer coeff"=w261:dbl[], "Zer index (starting from 3)"=w262:dbl[])  [unwired: 7 in]
                      "Initial Zer index (starting from 4)\nrandomly generated" <- w262
                      "Initial Zer coeff\nRandomly generated" <- w261
                    }
                  }
                }
                frame #1 {
                  # "read in offset command"
                  n64 = call-poly <vilib>:"Read From Spreadsheet File.vi"("format (%.3f)"="%.8f", "file path (dialog if empty)"="Offset command file") -> ("first row"=w265:dbl[])  [unwired: 5 in, 4 out]
                }
                frame #2 {
                  w290 = 0.0
                  # "ini zern coeff"
                  # "offset+ini command"
                  # "Zern coeff"
                  # "Zern index"
                  # "calculate the command:\nfor phase diversity"
                  n65 = Array Size(array="Zern index in 2") -> (size(s)=w288:i32)
                  n66 = call-poly <vilib>:"Ramp Pattern.vi"("start"=w290, "end"=w290, "samples"=w288) -> ("Ramp Pattern"=w287:dbl[])  [unwired: 7 in, 1 out]
                  n67 = Build Array(w287, "Zern index in 2", "Zern index in 3", "Zern index in 4", "Zern index in 5") -> (w272:T5)
                  n68 = Build Array(w287, "Zern coef in 2", "Zern coef in 3", "Zern coef in 4", "Zern coef in 5") -> (w291:T5)
                  n69 = Transpose Matrix(1:w291) -> (0:w284:T5)
                  n70 = Transpose Matrix(1:w272) -> (0:w282:T5)
                  n71 = Array Size(array=w272) -> (size(s)=w273:i32[])
                  n72 = Index Array(array=w273, index=1) -> (element=w281:i32)
                  "# of Phase" <- w281
                  n73 = stacked-sequence {
                    seq-local: [w300 _ _] -> [_ w318 w384]
                    seq-local: [w301 _ _] -> [_ w312 _]
                    seq-local: [_ w311 _] -> [_ _ w381]
                    seq-local: [w299 _ _] -> [_ w310 _]
                    tunnel: w281 -> [_ w323 _]
                    tunnel: w271 -> [w308 _ _]
                    tunnel: w270 -> [w307 w313 _]
                    tunnel: w276 -> [w306 w320 _]
                    tunnel: w285 -> [w304 _ _]
                    tunnel: w282 -> [_ w322 _]
                    tunnel: w284 -> [_ w321 _]
                    tunnel: w277 -> [w303 w319 _]
                    tunnel: [_ w317 _] -> w283
                    tunnel: w280 -> [_ w315 w382]
                    tunnel: w279 -> [_ w316 w383]
                    tunnel: w278 -> [_ w314 _]
                    tunnel: w275 -> [w302 _ _]
                    tunnel: [_ _ w380] -> w274
                    tunnel: [w300 _ _] -> w269
                    tunnel: w268 -> [_ w309 w378]
                    frame #0 {
                      n74 = call "zern2command_test.vi"("Initial haso file"=w303, "error in (no error)"=w302, "interaction matrix file"=w306, "Zern coef in"=w307, "Zern index in"=w308) -> ("error out"=w301:errorcluster, "Zern coef out"=w299:sgl[], "Offset positions"=w305:sgl[])  [unwired: 4 in]
                      n75 = Add(x=w305, y=w304) -> (x+y=w300:dbl[])
                    }
                    frame #1 {
                      n76 = for {
                        N: w323 -> [w326]
                        tunnel: w322 -> [w339] mode=indexing
                        tunnel: w321 -> [w338] mode=indexing
                        tunnel: w320 -> [w337]
                        tunnel: w319 -> [w336]
                        tunnel: w318 -> [w335]
                        tunnel: [w334] -> w317 mode=indexing
                        tunnel: w316 -> [w333]
                        tunnel: w315 -> [w332]
                        tunnel: w314 -> [w331]
                        tunnel: w313 -> [w330]
                        tunnel: w312 -> [w329]
                        tunnel: [w328] -> w311
                        tunnel: w310 -> [w325]
                        tunnel: w309 -> [w324]
                        i -> [w327]
                        n77 = stacked-sequence {
                          seq-local: [w345 _] -> [_ w364]
                          seq-local: [w341 _] -> [_ w363]
                          tunnel: w339 -> [w354 _]
                          tunnel: w338 -> [w353 _]
                          tunnel: w337 -> [w352 _]
                          tunnel: w336 -> [w351 _]
                          tunnel: w335 -> [w349 _]
                          tunnel: [w348 _] -> w334
                          tunnel: w333 -> [_ w366]
                          tunnel: w332 -> [_ w365]
                          tunnel: w331 -> [_ _]
                          tunnel: w327 -> [w347 _]
                          tunnel: w330 -> [w343 _]
                          tunnel: w329 -> [w342 _]
                          tunnel: [_ w362] -> w328
                          tunnel: w327 -> [_ _]
                          tunnel: w326 -> [_ _]
                          tunnel: w325 -> [w340 _]
                          tunnel: w324 -> [_ w359]
                          frame #0 {
                            n78 = Equal To 0?(x=w347) -> (x = 0?=w346:bool)
                            n79 = call "zern2command_test.vi"("Initial haso file"=w351, "error in (no error)"=w342, "interaction matrix file"=w352, "Zern coef in"=w353, "Zern index in"=w354) -> ("error out"=w341:errorcluster, "Zern coef out"=w344:sgl[], "Offset positions"=w350:sgl[])  [unwired: 4 in]
                            n80 = case shown="False" w346 {
                              tunnel: [w355 w356] -> w345
                              tunnel: w344 -> [w355 _]
                              tunnel: w343 -> [_ _]
                              tunnel: w340 -> [_ w356]
                              frame False {
                              }
                              frame True {
                              }
                            }
                            n81 = Add(x=w349, y=w350) -> (x+y=w348:dbl[])
                          }
                          frame #1 {
                            n82 = Number To Fractional String(number=w359, precision (6)=0) -> (F-format string=w358:string)  [unwired: 2 in]
                            n83 = Concatenate Strings(w366, w365, "_", w358, "_coeff.txt") -> (w374:string)
                            n84 = String To Path(string=w374) -> (path=w373:path)
                            n85 = Open/Create/Replace File(file path (use dialog)=w373, error in=w363, operation (0:open)=3) -> (refnum out=w370:refnum<file>, error out=w371:errorcluster)  [unwired: 3 in, 1 out]
                            n86 = Array To Spreadsheet String(array=w364, 3:"%f") -> (spreadsheet string=w361:string)  [unwired: 1 in]
                            n87 = Set File Position(refnum=w370, from (0:start)=1, error in=w371) -> (refnum out=w368:refnum<file>, error out=w367:errorcluster)  [unwired: 1 in]
                            n88 = Write to Text File(file (use dialog)=w368, text=w361, error in=w367) -> (error out=w362:errorcluster)  [unwired: 1 in, 2 out]
                          }
                        }
                      }
                    }
                    frame #2 {
                      n89 = Number To Fractional String(number=w378, precision (6)=0) -> (F-format string=w377:string)  [unwired: 2 in]
                      n90 = Concatenate Strings(w383, w382, "_", w377, "_IniAbr+offset.txt") -> (w393:string)
                      n91 = String To Path(string=w393) -> (path=w391:path)
                      n92 = Open/Create/Replace File(file path (use dialog)=w391, error in=w381, operation (0:open)=3) -> (refnum out=w388:refnum<file>, error out=w389:errorcluster)  [unwired: 3 in, 1 out]
                      n93 = Array To Spreadsheet String(array=w384, 3:"%f") -> (spreadsheet string=w395:string)  [unwired: 1 in]
                      n94 = Set File Position(refnum=w388, from (0:start)=1, error in=w389) -> (refnum out=w386:refnum<file>, error out=w385:errorcluster)  [unwired: 1 in]
                      n95 = Write to Text File(file (use dialog)=w386, text=w395, error in=w385) -> (error out=w380:errorcluster)  [unwired: 1 in, 2 out]
                    }
                  }
                }
                frame #3 {
                  # "set andor kinetics and spooling, \nstart acquire and wait for the external trigger"
                  n96 = Number To Fractional String(number=w399, precision (6)=0) -> (F-format string=w397:string)  [unwired: 2 in]
                  n97 = Concatenate Strings(w403, w402, "_PhsDiv_ToBeDeleted_", w397) -> (w400:string)
                  n98 = call "SetSpool_WaitForExtTrigger.vi"("path and name"=w400, "Kinetic Series"=w404) -> ()  [unwired: 10 in]
                }
                frame #4 {
                  # "take phase diversity pictures"
                  n99 = for {
                    N: w411 -> [_]
                    tunnel: w416 -> [w427]
                    tunnel: w415 -> [w426]
                    tunnel: w414 -> [w425]
                    tunnel: w410 -> [w424]
                    tunnel: w413 -> [w423]
                    tunnel: w412 -> [w422] mode=indexing
                    tunnel: w409 -> [w421]
                    tunnel: w408 -> [w420]
                    tunnel: [w419] -> w406
                    tunnel: [w418] -> w407
                    tunnel: w405 -> [w417]
                    n100 = stacked-sequence {
                      seq-local: [w428 _] -> [_ w438]
                      tunnel: w427 -> [_ w435]
                      tunnel: w426 -> [_ _]
                      tunnel: w425 -> [_ _]
                      tunnel: w424 -> [_ _]
                      tunnel: w423 -> [_ _]
                      tunnel: w422 -> [w429 _]
                      tunnel: w421 -> [_ w439]
                      tunnel: w420 -> [w430 _]
                      tunnel: [_ w437] -> w419
                      tunnel: [_ w436] -> w418
                      tunnel: w417 -> [w431 _]
                      frame #0 {
                        # "response time of mirror"
                        n101 = call <userlib>:"LVClass_WavefrontCorrector Move to Absolute Position.vi"("WavefrontCorrector in"=w431, "Absolute Positions"=w429, "error in (no error)"=w430) -> ("error out"=w428:errorcluster)  [unwired: 11 in, 1 out]
                        n102 = Add(x=5, y=10) -> (x+y=w432:i32)
                        n103 = Wait (ms)(milliseconds to wait=w432) -> ()  [unwired: 1 out]
                      }
                      frame #1 {
                        n104 = for {
                          N: w435 -> [_]
                          tunnel: w439 -> [w444]
                          tunnel: w438 -> [w443]
                          tunnel: [w442] -> w437
                          tunnel: [w441] -> w436
                          tunnel: w435 -> [w440]
                          n105 = stacked-sequence {
                            tunnel: w444 -> [w449 _]
                            tunnel: w443 -> [w447 _]
                            tunnel: [w446 _] -> w442
                            tunnel: [w445 _] -> w441
                            tunnel: w440 -> [_ w454]
                            frame #0 {
                              n106 = local read "EMCCD trigger port"() -> (w452:tag)
                              n107 = Add(x=w449, y=0.04) -> (x+y=w448:dbl)
                              n108 = Multiply(x=w448, y=1000.0) -> (x*y=w445:dbl)
                              n109 = call "trig EMCCD.vi"("error in (no error)"=w447, "exp time (ms)"=w445, "lines"=w452) -> ("error out"=w446:errorcluster)
                            }
                            frame #1 {
                              n110 = Not Equal?(x=w454, y=1) -> (x != y?=w455:bool)
                              n111 = case shown="True" w455 {
                                frame False {
                                }
                                frame True {
                                n112 = Wait (ms)(milliseconds to wait=50) -> ()  [unwired: 1 out]
                                }
                              }
                            }
                          }
                        }
                      }
                    }
                  }
                }
                frame #5 {
                  # "send out a trigger to EMCCD to end the aquisition."
                  n113 = local read "EMCCD trigger port"() -> (w458:tag)
                  n114 = call "trig EMCCD.vi"("exp time (ms)"=w457, "lines"=w458) -> ()  [unwired: 1 in, 1 out]
                }
                frame #6 {
                  w465 = 0
                  # "save phase diversity pictures:\npictures per phase*number of phases (Eg: 2*5=10 pictures in this file)"
                  n115 = Number To Fractional String(number=w469, precision (6)=w465) -> (F-format string=w464:string)  [unwired: 2 in]
                  n116 = Concatenate Strings(w470, "_", w464) -> (w460:string)
                  "phase diversity file name" <- w460
                  n117 = Concatenate Strings(w460, ".tif") -> (w461:string)
                  n118 = Concatenate Strings(w468, w461) -> (w463:string)
                  n119 = call <userlib>:"SaveAsTiff.vi"("path"=w463, "palette"="C:\\Program Files\\Andor SOLIS\\GREY.PAL", "position"=w465, "type"=1) -> ()  [unwired: 10 in, 2 out]
                }
                frame #7 {
                  # "offset+ini path and name no.tif"
                  # "groundtruth path and name no.tif"
                  # "take a picture of groundtruth and offset+ini abbr, and cal imq for each"
                  n120 = stacked-sequence {
                    seq-local: [w482 _ _ _] -> [_ w495 _ _]
                    seq-local: [_ _ w498 _] -> [_ _ _ w511]
                    tunnel: w480 -> [w487 _ w504 _]
                    tunnel: w479 -> [w486 _ w503 _]
                    tunnel: w478 -> [w485 _ w502 _]
                    tunnel: w477 -> [w484 _ w501 _]
                    tunnel: w474 -> [_ _ w500 _]
                    tunnel: w476 -> [w483 _ w499 _]
                    tunnel: w475 -> [_ w496 _ w514]
                    tunnel: [_ w492 _ _] -> w473
                    tunnel: w472 -> [w481 _ _ _]
                    tunnel: [_ _ _ w509] -> w471
                    frame #0 {
                      # "take a picture of groundtruth"
                      n121 = Number To Fractional String(number=w485, precision (6)=0) -> (F-format string=w488:string)  [unwired: 2 in]
                      n122 = Concatenate Strings(w487, w486, "_grdtrth_", w488) -> (w482:string)
                      n123 = call "Apply DM command and take picture.vi"("WavefrontCorrector in"=w483, "Offset positions"=w481, "trigger time (ms)"=w484, "# of pictures"=1, "path and file name, no .tif at the end"=w482) -> ()  [unwired: 6 in, 1 out]
                    }
                    frame #1 {
                      # "calculate imq of groundtruth"
                      n124 = Concatenate Strings(w495, ".tif") -> (w493:string)
                      n125 = call "MATLAB image quality metrics.vi"("Background Value"=w496, "File Path and Name w/.tif"=w493, "Metrics Type"="Metrics Type") -> ("image quality"=w492:dbl)  [unwired: 8 in]
                    }
                    frame #2 {
                      # "take a picture of offset+ini abbr"
                      n126 = Number To Fractional String(number=w502, precision (6)=0) -> (F-format string=w505:string)  [unwired: 2 in]
                      n127 = Concatenate Strings(w504, w503, "_abbr_", w505) -> (w498:string)
                      n128 = call "Apply DM command and take picture.vi"("WavefrontCorrector in"=w499, "Offset positions"=w500, "trigger time (ms)"=w501, "# of pictures"=1, "path and file name, no .tif at the end"=w498) -> ()  [unwired: 6 in, 1 out]
                    }
                    frame #3 {
                      # "calculate imq of offset+ini"
                      n129 = local read "Metrics Type"() -> (w510:T3)
                      n130 = Concatenate Strings(w511, ".tif") -> (w512:string)
                      n131 = call "MATLAB image quality metrics.vi"("Background Value"=w514, "File Path and Name w/.tif"=w512, "Metrics Type"=w510) -> ("image quality"=w509:dbl)  [unwired: 8 in]
                    }
                  }
                }
                frame #8 {
                  # "run matlab correction?"
                  n132 = case shown="True" w528 {
                    tunnel: w533 -> [_ w556]
                    tunnel: w534 -> [_ w555]
                    tunnel: w532 -> [_ w554]
                    tunnel: w531 -> [_ w553]
                    tunnel: w518 -> [_ w552]
                    tunnel: w530 -> [_ w551]
                    tunnel: w529 -> [_ w550]
                    tunnel: w517 -> [_ w549]
                    tunnel: w527 -> [_ _]
                    tunnel: [0 w548] -> w526
                    tunnel: w525 -> [_ w547]
                    tunnel: [errorcluster {"status"=FALSE, "code"=0, "source"=""} ("Error out 2") w546] -> w524
                    tunnel: w523 -> [_ w545]
                    tunnel: w522 -> [_ w544]
                    tunnel: w521 -> [_ _]
                    tunnel: w520 -> [_ w543]
                    tunnel: w519 -> [_ w540]
                    tunnel: w518 -> [_ w542]
                    tunnel: w517 -> [_ w541]
                    tunnel: w516 -> [_ w538]
                    tunnel: w515 -> [_ w537]
                    frame False {
                    }
                    frame True {
                      # "matlab reconstructed Zern"
                      n133 = stacked-sequence {
                        seq-local: [w569 _ _ _ _ _ _ _ _ _ _] -> [_ _ _ _ _ _ w711 _ _ _ _]
                        seq-local: [w571 _ _ _ _ _ _ _ _ _ _] -> [_ _ _ _ _ _ w707 _ _ _ _]
                        seq-local: [_ _ _ _ w690 _ _ _ _ _ _] -> [_ _ _ _ _ w697 _ _ _ _ _]
                        seq-local: [_ _ w678 _ _ _ _ _ _ _ _] -> [_ _ _ w685 _ _ _ _ _ _ _]
                        seq-local: [_ _ _ w687 _ _ _ _ _ _ _] -> [_ _ _ _ w691 _ _ _ _ _ _]
                        seq-local: [_ w670 _ _ _ _ _ _ _ _ _] -> [_ _ _ _ _ _ _ _ _ _ w745]
                        tunnel: w556 -> [w570 w673 _ _ _ _ _ _ _ w734 _]
                        tunnel: w555 -> [w568 w672 _ _ _ _ _ _ _ w733 _]
                        tunnel: w554 -> [w560 _ _ _ _ _ w710 _ _ _ _]
                        tunnel: w553 -> [w563 _ _ _ w692 _ w709 _ _ _ _]
                        tunnel: w552 -> [_ _ _ w689 _ w699 _ w717 w731 _ _]
                        tunnel: w550 -> [_ _ w679 _ _ _ _ _ _ _ _]
                        tunnel: [_ _ _ w688 _ _ _ _ _ _ _] -> _
                        tunnel: w551 -> [_ _ _ w688 _ _ _ w716 _ _ _]
                        tunnel: w549 -> [w567 w671 _ _ _ _ _ _ _ w735 _]
                        tunnel: [w566 _ _ _ _ _ _ _ _ _ _] -> w548
                        tunnel: w547 -> [_ _ w680 _ _ _ _ _ _ _ _]
                        tunnel: [_ _ _ _ _ _ _ w715 _ _ _] -> w546
                        tunnel: w545 -> [w557 _ w681 _ w693 _ w703 _ _ _ _]
                        tunnel: w544 -> [_ w674 _ _ _ _ _ _ _ _ w743]
                        tunnel: w543 -> [w565 _ _ _ _ _ _ _ _ _ _]
                        tunnel: w542 -> [w562 _ _ _ _ _ _ _ _ _ _]
                        tunnel: w541 -> [w561 _ _ _ _ _ _ _ _ _ _]
                        tunnel: 2 -> [w564 _ _ _ _ _ _ _ _ _ _]
                        tunnel: w540 -> [w559 _ _ _ _ _ _ _ _ _ _]
                        tunnel: w538 -> [w558 _ _ _ _ _ _ _ _ _ _]
                        tunnel: w537 -> [_ _ _ _ _ _ w700 _ _ _ _]
                        frame #0 {
                          n134 = while {
                            tunnel: [w590] -> w571
                            tunnel: w570 -> [w589]
                            tunnel: [w588] -> w569
                            tunnel: w568 -> [w587]
                            tunnel: w567 -> [w586]
                            tunnel: [w585] -> w566
                            tunnel: w565 -> [w584]
                            shift-right: [w575] -> _
                            shift-left: w564 -> [w583]
                            tunnel: w563 -> [w582]
                            tunnel: w562 -> [w581]
                            tunnel: w561 -> [w580]
                            tunnel: w560 -> [w579]
                            tunnel: w559 -> [w578]
                            tunnel: w558 -> [w573]
                            tunnel: w557 -> [w572]
                            stop <- w576 stop-if-true
                            n135 = stacked-sequence {
                              seq-local: [w599 _ _ _] -> [_ w633 _ _]
                              seq-local: [_ w635 _ _] -> [_ _ w650 _]
                              seq-local: [w598 _ _ _] -> [_ w632 _ _]
                              tunnel: [w598 _ _ _] -> w590
                              tunnel: w589 -> [w618 w636 _ _]
                              tunnel: [w599 _ _ _] -> w588
                              tunnel: w587 -> [w595 w634 _ _]
                              tunnel: w586 -> [w612 _ _ _]
                              tunnel: [w602 _ _ _] -> w585
                              tunnel: w584 -> [w600 _ w651 _]
                              tunnel: w583 -> [w597 w628 _ w664]
                              tunnel: w582 -> [_ w631 _ _]
                              tunnel: w581 -> [_ w630 _ _]
                              tunnel: w580 -> [_ w629 _ _]
                              tunnel: w579 -> [_ w627 _ _]
                              tunnel: w578 -> [_ _ w649 _]
                              tunnel: [_ _ w648 _] -> w577
                              tunnel: [_ _ _ w659] -> w575
                              tunnel: [_ _ _ w656] -> w574
                              tunnel: w573 -> [_ w626 _ _]
                              tunnel: w572 -> [_ w625 _ _]
                              frame #0 {
                                w592 = "_"
                                # "MATLAB does the reconstruction, written by Min Guo"
                                # "other parameters are default in this VI"
                                n136 = Number To Fractional String(number=w612, precision (6)=0) -> (F-format string=w591:string)  [unwired: 2 in]
                                n137 = Concatenate Strings(w595, "_", w591) -> (w601:string)
                                n138 = String To Path(string=w618) -> (path=w619:path)
                                n139 = Number To Fractional String(number=w597, precision (6)=0) -> (F-format string=w594:string)  [unwired: 2 in]
                                n140 = Concatenate Strings(w618, w595, w592, w594, "ImgCorr", w592, w591) -> (w617:string)
                                n141 = String To Path(string=w617) -> (path=w616:path)
                                n142 = call "recon_zern_fileIO_MATLAB_v2.vi"("Number of Phase"=w597, "Number for average"="Number for average", "Crop Size of image"="Crop Size of image", "Background Value"=w600, "Zernike Order"="Zernike Order", "Use GPU"="Use GPU", "Iteration Number"="Iteration Number", "File Name"=w601, "Gamma Value"="Gamma Value", "Path In"=w619, "Show Input"="Show Input", "Path Out"=w616, "Show Recon"="Show Recon") -> ("Zern coef out"=w614:sgl[], "RMSE Value"=w602:dbl, "error out"=w598:errorcluster)  [unwired: 3 in, 1 out]
                                n143 = case shown="True" "Keep Reconstructed Defocus component?" {
                                tunnel: w614 -> [w620 w624]
                                tunnel: [w620 w621] -> w599
                                frame False {
                                }
                                frame True {
                                n144 = Replace Array Subset(array=w624, new element=0.0, index=2) -> (w621:sgl[])
                                }
                                }
                              }
                              frame #1 {
                                w638 = 0
                                w647 = 1
                                # "get correction command\ntake a picture"
                                n145 = call-poly <vilib>:"Ramp Pattern.vi"("start"=w647, "end"=32, "delta"=w647) -> ("Ramp Pattern"=w645:dbl[])  [unwired: 6 in, 2 out]
                                n146 = call "zern2command_test.vi"("Initial haso file"=w626, "error in (no error)"=w632, "interaction matrix file"=w627, "Zern coef in"=w633, "Zern index in"=w645) -> ("Offset positions"=w644:sgl[])  [unwired: 4 in, 2 out]
                                n147 = Add(x=w631, y=w644) -> (x+y=w643:dbl[])
                                n148 = Number To Fractional String(number=w629, precision (6)=w638) -> (F-format string=w640:string)  [unwired: 2 in]
                                n149 = Number To Fractional String(number=w628, precision (6)=w638) -> (F-format string=w637:string)  [unwired: 2 in]
                                n150 = Concatenate Strings(w636, w634, "_", w637, "ImgCorr_", w640) -> (w635:string)
                                n151 = call "Apply DM command and take picture.vi"("WavefrontCorrector in"=w625, "Offset positions"=w643, "trigger time (ms)"=w630, "# of pictures"=1, "path and file name, no .tif at the end"=w635) -> ()  [unwired: 6 in, 1 out]
                              }
                              frame #2 {
                                n152 = local read "Metrics Type"() -> (w653:T3)
                                n153 = Concatenate Strings(w650, ".tif") -> (w654:string)
                                n154 = call "MATLAB image quality metrics.vi"("Background Value"=w651, "File Path and Name w/.tif"=w654, "Metrics Type"=w653) -> ("image quality"=w652:dbl)  [unwired: 8 in]
                                n155 = Greater?(x=w652, y=w649) -> (0:w648:bool)
                              }
                              frame #3 {
                                n156 = Equal?(x="number of phase div image", y=0.9) -> (x = y?=w660:bool)
                                n157 = To Byte Integer(number="number of phase div image") -> (8bit integer=w663:i8)
                                n158 = Add(x=w664, y=w663) -> (x+y=w659:i32)
                                n159 = case shown="False" w660 {
                                tunnel: w659 -> [_ w668]
                                tunnel: [FALSE w667] -> w657
                                frame False {
                                }
                                frame True {
                                n160 = Greater?(x=w668, y=3) -> (0:w667:bool)
                                }
                                }
                                n161 = Greater?(x=w659, y=5) -> (0:w658:bool)
                                n162 = Or(x=w658, y=w657) -> (x .or. y?=w656:bool)
                              }
                            }
                            n163 = Or(x=w577, y=w574) -> (x .or. y?=w576:bool)
                          }
                        }
                        frame #1 {
                          # "set andor kinetics and spooling, \nstart acquire and wait for the external trigger"
                          n164 = Number To Fractional String(number=w671, precision (6)=0) -> (F-format string=w675:string)  [unwired: 2 in]
                          n165 = Concatenate Strings(w673, w672, "_Corr_ToBeDeleted_", w675) -> (w670:string)
                          n166 = call "SetSpool_WaitForExtTrigger.vi"("path and name"=w670, "Kinetic Series"=w674) -> ()  [unwired: 10 in]
                        }
                        frame #2 {
                          # "groundtruth command"
                          # "response time of mirror"
                          n167 = call <userlib>:"LVClass_WavefrontCorrector Move to Absolute Position.vi"("WavefrontCorrector in"=w681, "Absolute Positions"=w680, "error in (no error)"=w679) -> ("error out"=w678:errorcluster)  [unwired: 11 in, 1 out]
                          n168 = Add(x=5, y=10) -> (x+y=w682:i32)
                          n169 = Wait (ms)(milliseconds to wait=w682) -> ()  [unwired: 1 out]
                        }
                        frame #3 {
                          # "take offset/groundtruth picture, only one"
                          n170 = local read "EMCCD trigger port"() -> (w686:tag)
                          n171 = call "trig EMCCD.vi"("error in (no error)"=w685, "exp time (ms)"=w689, "lines"=w686) -> ("error out"=w687:errorcluster)
                        }
                        frame #4 {
                          # "aberrated picture command"
                          # "response time of mirror"
                          n172 = call <userlib>:"LVClass_WavefrontCorrector Move to Absolute Position.vi"("WavefrontCorrector in"=w693, "Absolute Positions"=w692, "error in (no error)"=w691) -> ("error out"=w690:errorcluster)  [unwired: 11 in, 1 out]
                          n173 = Add(x=5, y=10) -> (x+y=w694:i32)
                          n174 = Wait (ms)(milliseconds to wait=w694) -> ()  [unwired: 1 out]
                        }
                        frame #5 {
                          # "take offset+initial aberr picture, only one"
                          n175 = local read "EMCCD trigger port"() -> (w698:tag)
                          n176 = call "trig EMCCD.vi"("error in (no error)"=w697, "exp time (ms)"=w699, "lines"=w698) -> ()  [unwired: 1 out]
                        }
                        frame #6 {
                          w714 = 1
                          # "correction command"
                          # "response time of mirror"
                          n177 = call-poly <vilib>:"Ramp Pattern.vi"("start"=w714, "end"=32, "delta"=w714) -> ("Ramp Pattern"=w712:dbl[])  [unwired: 6 in, 2 out]
                          n178 = call "zern2command_test.vi"("Initial haso file"=w700, "error in (no error)"=w707, "interaction matrix file"=w710, "Zern coef in"=w711, "Zern index in"=w712) -> ("error out"=w701:errorcluster, "Offset positions"=w708:sgl[])  [unwired: 4 in, 1 out]
                          n179 = Add(x=w709, y=w708) -> (x+y=w702:dbl[])
                          n180 = call <userlib>:"LVClass_WavefrontCorrector Move to Absolute Position.vi"("WavefrontCorrector in"=w703, "Absolute Positions"=w702, "error in (no error)"=w701) -> ()  [unwired: 11 in, 2 out]
                          n181 = Add(x=5, y=10) -> (x+y=w704:i32)
                          n182 = Wait (ms)(milliseconds to wait=w704) -> ()  [unwired: 1 out]
                        }
                        frame #7 {
                          # "corrected pictures"
                          n183 = for {
                            N: w716 -> [w718]
                            tunnel: w717 -> [w721]
                            shift-right: [w719] -> w715
                            shift-left: _ -> [w720]
                            n184 = stacked-sequence {
                              tunnel: w721 -> [w724 _]
                              tunnel: w720 -> [w723 _]
                              tunnel: [w722 _] -> w719
                              tunnel: w718 -> [_ w726]
                              frame #0 {
                                n185 = local read "EMCCD trigger port"() -> (w725:tag)
                                n186 = call "trig EMCCD.vi"("error in (no error)"=w723, "exp time (ms)"=w724, "lines"=w725) -> ("error out"=w722:errorcluster)
                              }
                              frame #1 {
                                n187 = Not Equal?(x=w726, y=1) -> (x != y?=w728:bool)
                                n188 = case shown="True" w728 {
                                frame False {
                                }
                                frame True {
                                n189 = Wait (ms)(milliseconds to wait=50) -> ()  [unwired: 1 out]
                                }
                                }
                              }
                            }
                          }
                        }
                        frame #8 {
                          # "one more trigger to end picture acquisition"
                          n190 = local read "EMCCD trigger port"() -> (w730:tag)
                          n191 = call "trig EMCCD.vi"("exp time (ms)"=w731, "lines"=w730) -> ()  [unwired: 1 in, 1 out]
                        }
                        frame #9 {
                          w738 = 0
                          # "save:\none groundtruth picture\none offset+abrr picture\nPictures per phase*corrected picture"
                          n192 = Number To Fractional String(number=w735, precision (6)=w738) -> (F-format string=w737:string)  [unwired: 2 in]
                          n193 = Concatenate Strings(w733, "_grdtrth_abrr_Corr_", w737, ".tif") -> (w742:string)
                          "Corrected Picture name" <- w742
                          n194 = Concatenate Strings(w734, w742) -> (w736:string)
                          n195 = call <userlib>:"SaveAsTiff.vi"("path"=w736, "palette"="C:\\Program Files\\Andor SOLIS\\GREY.PAL", "position"=w738, "type"=1) -> ()  [unwired: 10 in, 2 out]
                        }
                        frame #10 {
                          n196 = case shown="True" TRUE {
                            tunnel: w745 -> [_ w747]
                            tunnel: w743 -> [_ w746]
                            frame False {
                            }
                            frame True {
                              # "delete spooling data"
                              n197 = for {
                                N: w746 -> [_]
                                tunnel: w747 -> [w754]
                                i -> [w752]
                                n198 = Number To Fractional String(number=w752, precision (6)=0) -> (F-format string=w750:string)  [unwired: 2 in]
                                n199 = Concatenate Strings(w754, "000000000", w750, ".dat") -> (w749:string)
                                n200 = String To Path(string=w749) -> (path=w755:path)
                                n201 = Delete(path (use dialog)=w755) -> ()  [unwired: 4 in, 3 out]
                              }
                            }
                          }
                        }
                      }
                    }
                  }
                }
                frame #9 {
                  # "delete spooling data of phase diversity"
                  n202 = case shown="True" TRUE {
                    tunnel: w758 -> [_ w760]
                    tunnel: w756 -> [_ w759]
                    frame False {
                    }
                    frame True {
                      n203 = for {
                        N: w759 -> [_]
                        tunnel: w760 -> [w766]
                        i -> [w764]
                        n204 = Greater?(x=w764, y=9) -> (0:w762:bool)
                        n205 = Number To Fractional String(number=w764, precision (6)=0) -> (F-format string=w768:string)  [unwired: 2 in]
                        n206 = case shown="False" w762 {
                          tunnel: ["000000000" "00000000"] -> w761
                          frame False {
                          }
                          frame True {
                          }
                        }
                        n207 = Concatenate Strings(w766, w761, w768, ".dat") -> (w765:string)
                        n208 = String To Path(string=w765) -> (path=w770:path)
                        n209 = Delete(path (use dialog)=w770) -> ()  [unwired: 4 in, 3 out]
                      }
                    }
                  }
                }
              }
            }
          }
          frame #2 {
            # "shut down shutter of 488nm laser"
            n210 = invoke class="MG17Motor" method="SC_Disable"(reference=w776, "lChanID"=w775) -> (reference out=w774:refnum<k7>, "lChanID"=w773:i32)  [unwired: 2 in, 2 out]
          }
          frame #3 {
            # "save the RMS of (calculated zer-real zer)"
            n211 = Concatenate Strings(w779, w778, "_RMSE.txt") -> (w784:string)
            n212 = String To Path(string=w784) -> (path=w783:path)
            n213 = Number To Fractional String(number=w780) -> (F-format string=w781:string[])  [unwired: 3 in]
            n214 = Write to Text File(file (use dialog)=w783, text=w781) -> (error out=w777:errorcluster)  [unwired: 2 in, 2 out]
          }
        }
        n215 = Merge Errors(w191, w190, w185) -> (w184:errorcluster)
        "Error out" <- w184
        n216 = Unbundle(w184) -> ("status"=w180:bool)  [unwired: 2 out]
        n217 = case shown="True" w180 {
          tunnel: [w206 w207] -> w183
          tunnel: w180 -> [w205 w207]
          frame False {
            n218 = Not(x=w205) -> (.not. x?=w206:bool)
          }
          frame True {
          }
        }
        n219 = Or(x=w183, y="?") -> (x .or. y?=w181:bool)
      }
    }
    frame #4 {
      n220 = case shown="True" "Turn off EMCCD when finished?" {
        frame False {
        }
        frame True {
          n221 = flat-sequence {
            frame #0 {
              n222 = call <userlib>:"CoolerOFF.vi"() -> ()  [unwired: 2 in, 2 out]
            }
            frame #1 {
              # "shut down EMCCD"
              n223 = call <userlib>:"ShutDown.vi"() -> ()  [unwired: 2 in, 2 out]
            }
          }
        }
      }
    }
    frame #5 {
      # "if not \"stop control\", the shutter can be control when the program is not running"
      # "shut down casao"
      n224 = call <userlib>:"LVClass_WavefrontCorrector dtor.vi"("WavefrontCorrector in"=w790, "error in (no error)"=w788) -> ("error out"=w787:errorcluster)  [unwired: 12 in, 1 out]
      n225 = call <userlib>:"LVClass_WavefrontCorrectorSet dtor.vi"("WavefrontCorrectorSet in"=w789, "error in (no error)"=w787) -> ()  [unwired: 12 in, 2 out]
      n226 = case shown="True" FALSE {
        tunnel: w791 -> [_ w792]
        frame False {
        }
        frame True {
          n227 = invoke class="MG17Motor" method="StopCtrl"(reference=w792) -> ()  [unwired: 2 in, 3 out]
        }
      }
    }
  }
